vi "Initialize Bus Monitor.vi"(8 "error in (no error)":errorcluster, 11 "IBusMonitor In":refnum<class "IBusMonitor.lvclass">) -> (0 "error out":errorcluster, 3 "IBusMonitor Out":refnum<class "IBusMonitor.lvclass">)   [LabVIEW 2018, in "MVA Framework.lvlib" / "MonitoredMediator.lvlib" / "IBusMonitor.lvclass"]
uses:
  IBusMonitor.lvclass
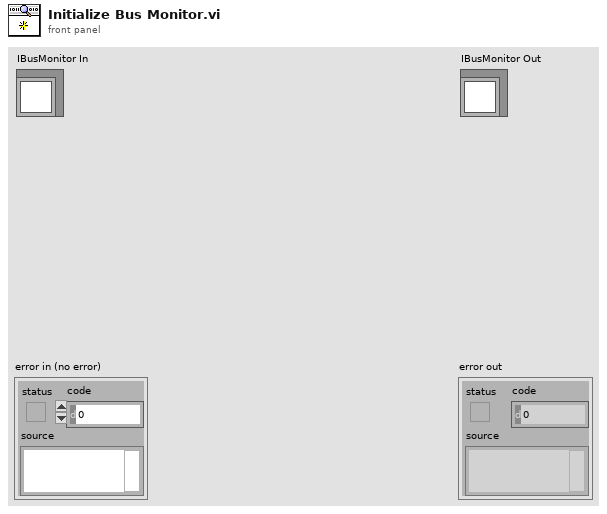
[diagram p1: front panel]
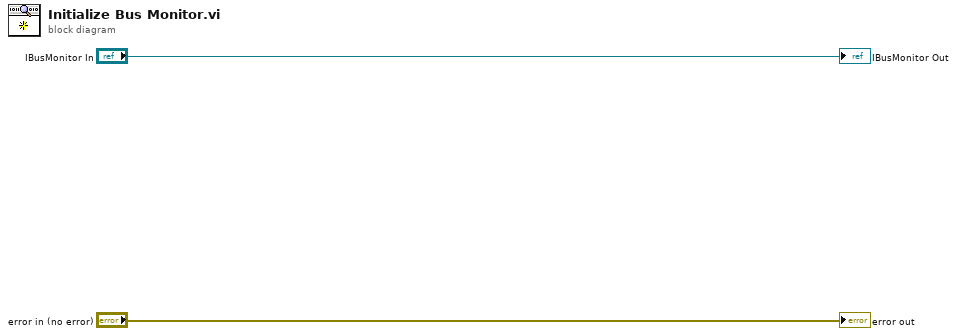
[diagram p0: block diagram]
diagram:
  "error out" <- "error in (no error)"
  "IBusMonitor Out" <- "IBusMonitor In"
